vi "New Results.vi"(8 "error in (no error)":errorcluster, 10 "Results":variant, 11 "POLARIS Target Focus Actor in":refnum<class "POLARIS Target Focus Actor.lvclass">) -> (0 "error out":errorcluster, 3 "POLARIS Target Focus Actor out":refnum<class "POLARIS Target Focus Actor.lvclass">)   [LabVIEW 2014, in "POLARIS Target Focus Actor.lvlib" / "POLARIS Target Focus Actor.lvclass"]
uses:
  POLARIS Target Focus Actor.lvclass
  POLARIS Target Focus Actor.lvclass/POLARIS Target Focus Actor.ctl
  <vilib>/ActorFramework/Message Enqueuer/Message Enqueuer.lvclass/Message Enqueuer.ctl
  <vilib>/ActorFramework/Message Enqueuer/Enqueue.vi
  <vilib>/ActorFramework/Message Priority Queue/Priority Enqueue.vi
  HIJ Vision Display/HIJ Vision Display Messages/Save Image Msg/Save Image Msg.lvclass
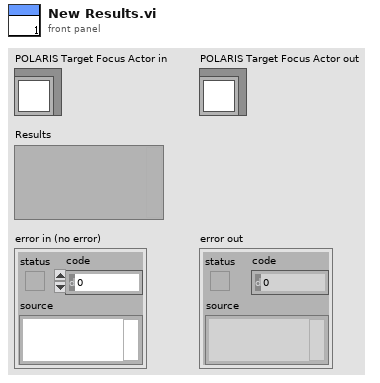
[diagram p1: front panel]
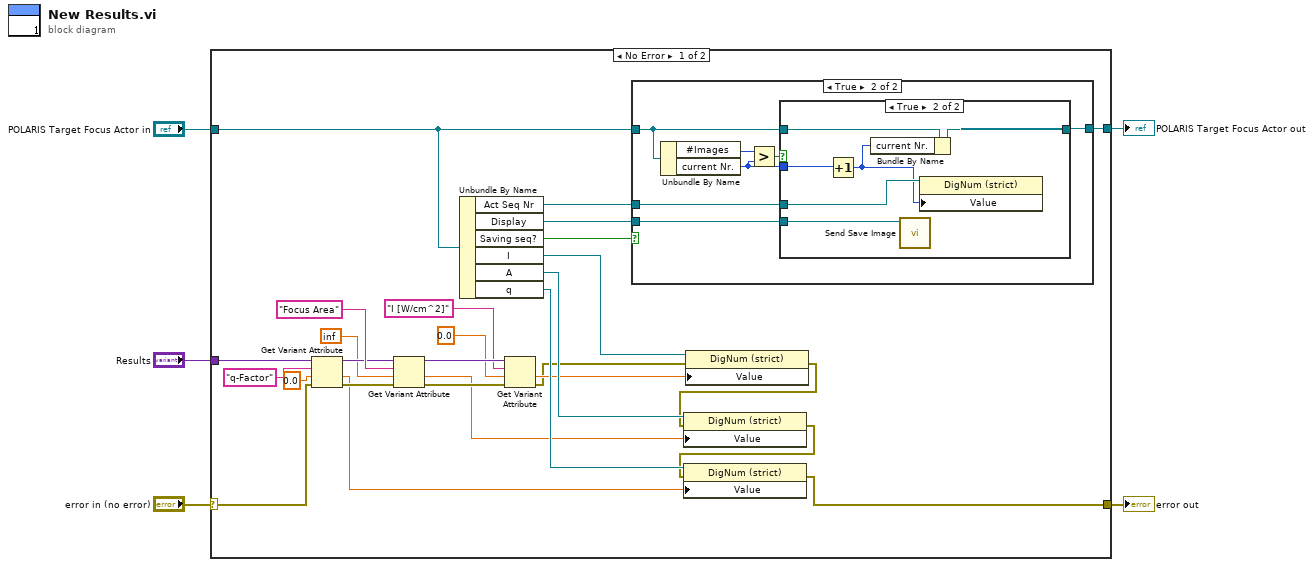
[diagram p0: block diagram]
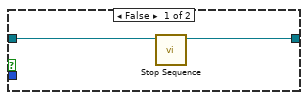
[diagram p3: hidden frame]
diagram:
  n1 = case shown="No Error" "error in (no error)" {
    selector: "error in (no error)" -> [w8 w50]
    tunnel: [w7 w50] -> w4
    tunnel: [w16 w49] -> w2
    tunnel: "POLARIS Target Focus Actor in" -> [w17 w49]
    tunnel: "Results" -> [w21 _]
    frame No Error {
      n2 = Get Variant Attribute(Variant=w21, name="q-Factor", default value (empty Variant)=0.0, error in=w8) -> (duplicate Variant=w29:variant, value=w14:dbl, error out=w25:errorcluster)  [unwired: 1 out]
      n3 = Get Variant Attribute(Variant=w29, name="Focus Area", default value (empty Variant)=inf, error in=w25) -> (duplicate Variant=w27:variant, value=w13:dbl, error out=w24:errorcluster)  [unwired: 1 out]
      n4 = Unbundle By Name(w17) -> ("Act Seq Nr"=w6:refnum<vi>, "Display"=w12:refnum<class "Message Enqueuer.lvclass">, "Saving seq?"=w15:bool, "I"=w32:refnum<vi>, "A"=w20:refnum<vi>, "q"=w19:refnum<vi>)
      n5 = Get Variant Attribute(Variant=w27, name="I [W/cm^2]", default value (empty Variant)=0.0, error in=w24) -> (value=w18:dbl, error out=w11:errorcluster)  [unwired: 2 out]
      n6 = case shown="True" w15 {
        tunnel: w17 -> [w33 w37]
        tunnel: [w33 w38] -> w16
        tunnel: w12 -> [_ w35]
        tunnel: w6 -> [_ w34]
        frame False {
        }
        frame True {
          n7 = Unbundle By Name(w37) -> ("#Images"=w40:u16, "current Nr."=w36:u16)
          n8 = Greater?(x=w40, y=w36) -> (0:w39:bool)
          n9 = case shown="True" w39 {
            tunnel: [w41 w47] -> w38
            tunnel: w37 -> [w42 w48]
            tunnel: w36 -> [_ w46]
            tunnel: w35 -> [_ w45]
            tunnel: w34 -> [_ w44]
            frame False {
              n10 = call "Stop Sequence.vi"("POLARIS Target Focus Actor in"=w42) -> ("POLARIS Target Focus Actor out"=w41:refnum<class "POLARIS Target Focus Actor.lvclass">)  [unwired: 9 in, 1 out]
            }
            frame True {
              n11 = Increment(x=w46) -> (x+1=w43:u16)
              n12 = Bundle By Name(cluster=w48, "current Nr."=w43) -> (w47:refnum<class "POLARIS Target Focus Actor.lvclass">)
              n13 = call "Send Save Image.vi"("Message Enqueuer"=w45) -> ()  [unwired: 9 in, 2 out]
              n14 = property class="DigNum (strict)"(reference=w44, "Value"=w43) -> ()  [unwired: 1 in, 2 out]
            }
          }
        }
      }
      n15 = property class="DigNum (strict)"(reference=w32, error in=w11, "Value"=w18) -> (error out=w10:errorcluster)  [unwired: 1 out]
      n16 = property class="DigNum (strict)"(reference=w20, error in=w10, "Value"=w13) -> (error out=w9:errorcluster)  [unwired: 1 out]
      n17 = property class="DigNum (strict)"(reference=w19, error in=w9, "Value"=w14) -> (error out=w7:errorcluster)  [unwired: 1 out]
    }
    frame Error {
    }
  }
  "error out" <- w4
  "POLARIS Target Focus Actor out" <- w2
